vi "System_Main.vi"() -> ()   [LabVIEW 2015, in "System.lvclass"]
uses:
  Classes/System/System.lvclass
  Classes/System/System.lvclass/System.ctl
  Classes/AssetInterface/Interface_Asset.lvclass
  Classes/DispatchInterface/Interface_Dispatch.lvclass
  Classes/TagBus/TagBus.lvclass
panel:
  out "Tag Values":dbl[](array[numeric])
  out "Tag Names":string[](array[string])
  in  "stop":bool
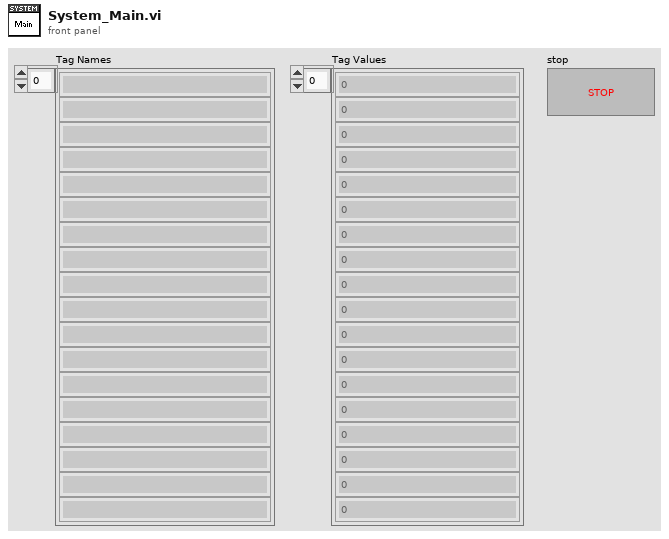
[diagram p1: front panel]
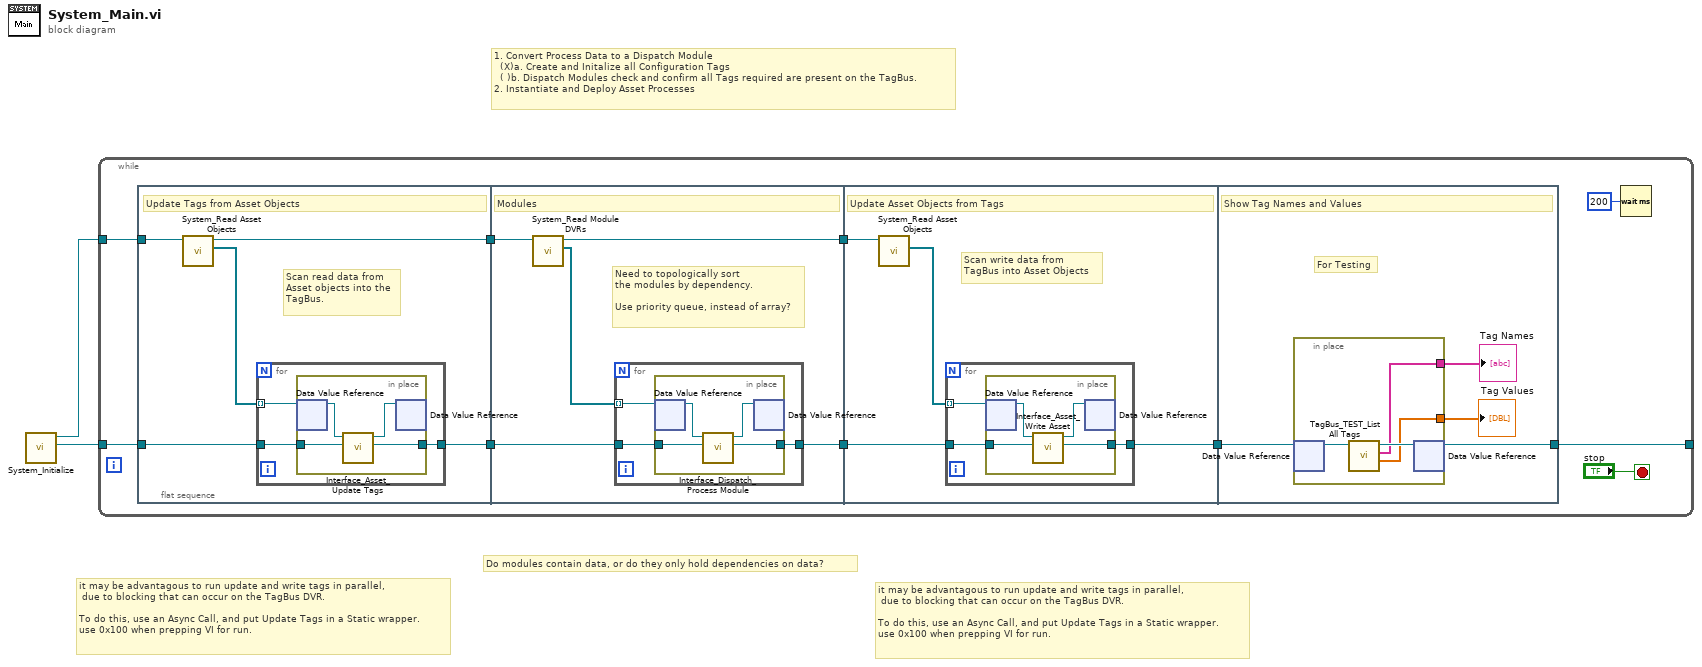
[diagram p0: block diagram]
diagram:
  # "Do modules contain data, or do they only hold dependencies on data?"
  # "it may be advantagous to run update and write tags in parallel,\n due to blocking that can occur on the TagBus DVR.\n\nTo do this, use an Async Call, and put Update Tags in a Static wrapper.\nuse 0x100 when prepping VI for run."
  # "it may be advantagous to run update and write tags in parallel,\n due to blocking that can occur on the TagBus DVR.\n\nTo do this, use an Async Call, and put Update Tags in a Static wrapper.\nuse 0x100 when prepping VI for run."
  # "1. Convert Process Data to a Dispatch Module\n  (X)a. Create and Initalize all Configuration Tags\n  ( )b. Dispatch Modules check and confirm all Tags required are present on the TagBus.\n2. Instantiate and Deploy Asset Processes"
  n1 = call "System_Initialize.vi"() -> ("TagBus DVR"=w1:refnum<data-value>, "System DVR out"=w2:refnum<data-value>)  [unwired: 10 in]
  n2 = while {
    tunnel: w1 -> [w8]
    tunnel: w2 -> [w10]
    tunnel: [w9] -> _
    stop <- "stop" stop-if-true
    n3 = flat-sequence {
      tunnel: w10 -> [w17]
      tunnel: [w15] -> w7
      tunnel: w8 -> [w14]
      tunnel: [w13] -> w6
      tunnel: w7 -> [w29]
      tunnel: [w28] -> w5
      tunnel: w6 -> [w26]
      tunnel: [w25] -> w4
      tunnel: w5 -> [w40]
      tunnel: w4 -> [w37]
      tunnel: [w38] -> w3
      tunnel: [w50] -> w9
      tunnel: w3 -> [w51]
      frame #0 {
        # "Scan read data from\nAsset objects into the\nTagBus."
        # "Update Tags from Asset Objects"
        n4 = call "System_Read Asset Objects.vi"("data value reference"=w17) -> ("Asset DVR Array"=w16:refnum<data-value>[], "data value reference out"=w15:refnum<data-value>)  [unwired: 9 in]
        n5 = for {
          tunnel: w16 -> [w18] mode=indexing
          tunnel: w14 -> [w20]
          tunnel: [w19] -> w13
          n6 = in-place {
            in-place-border: w20 -> [w24]
            in-place-border: [w23] -> w19
            n7 = in-place-dvr #1(w18) -> (w22:refnum<class "Interface_Asset.lvclass">)  [unwired: 1 out]
            n8 = call-dynamic "Interface_Asset_Update Tags.vi"("TagBus DVR"=w24, "Asset_Interface in"=w22) -> ("TagBus DVR out"=w23:refnum<data-value>, "Asset_Interface out"=w21:refnum<class "Interface_Asset.lvclass">)  [unwired: 7 in, 1 out]
            n9 = in-place-dvr #1(w21) -> ()  [unwired: 2 out]
          }
        }
      }
      frame #1 {
        # "Need to topologically sort\nthe modules by dependency.\n\nUse priority queue, instead of array?"
        # "Modules"
        n10 = call "System_Read Module DVRs.vi"("Data Value Reference in"=w29) -> ("Dispatch Module DVR Array"=w27:refnum<data-value>[], "Data Value Reference out"=w28:refnum<data-value>)  [unwired: 9 in]
        n11 = for {
          tunnel: w27 -> [w30] mode=indexing
          tunnel: w26 -> [w32]
          tunnel: [w31] -> w25
          n12 = in-place {
            in-place-border: w32 -> [w34]
            in-place-border: [w33] -> w31
            n13 = in-place-dvr #2(w30) -> (w36:refnum<class "Interface_Dispatch.lvclass">)  [unwired: 1 out]
            n14 = call-dynamic "Interface_Dispatch_Process Module.vi"("TagBus DVR"=w34, "Interface_Dispatch in"=w36) -> ("TagBus DVR out"=w33:refnum<data-value>, "Interface_Dispatch out"=w35:refnum<class "Interface_Dispatch.lvclass">)  [unwired: 7 in, 1 out]
            n15 = in-place-dvr #2(w35) -> ()  [unwired: 2 out]
          }
        }
      }
      frame #2 {
        # "Scan write data from\nTagBus into Asset Objects"
        # "Update Asset Objects from Tags"
        n16 = call "System_Read Asset Objects.vi"("data value reference"=w40) -> ("Asset DVR Array"=w39:refnum<data-value>[])  [unwired: 9 in, 1 out]
        n17 = for {
          tunnel: w39 -> [w41] mode=indexing
          tunnel: w37 -> [w43]
          tunnel: [w42] -> w38
          n18 = in-place {
            in-place-border: w43 -> [w45]
            in-place-border: [w44] -> w42
            n19 = in-place-dvr #3(w41) -> (w46:refnum<class "Interface_Asset.lvclass">)  [unwired: 1 out]
            n20 = call-dynamic "Interface_Asset_Write Asset.vi"("TagBus DVR"=w45, "Asset_Interface in"=w46) -> ("TagBus DVR out"=w44:refnum<data-value>, "Asset_Interface out"=w47:refnum<class "Interface_Asset.lvclass">)  [unwired: 7 in, 1 out]
            n21 = in-place-dvr #3(w47) -> ()  [unwired: 2 out]
          }
        }
      }
      frame #3 {
        # "For Testing"
        # "Show Tag Names and Values"
        n22 = in-place {
          in-place-border: [w53] -> w49
          in-place-border: [w52] -> w48
          n23 = in-place-dvr #4(w51) -> (w55:refnum<class "TagBus.lvclass">)  [unwired: 1 out]
          n24 = call "TagBus_TEST_List All Tags.vi"("TagBus in"=w55) -> ("values"=w52:dbl[], "Double"=w53:string[], "TagBus out"=w54:refnum<class "TagBus.lvclass">)  [unwired: 7 in, 1 out]
          n25 = in-place-dvr #4(w54) -> (w50:refnum<data-value>)  [unwired: 1 out]
        }
        "Tag Names" <- w49
        "Tag Values" <- w48
      }
    }
    n26 = Wait (ms)(milliseconds to wait=u32 200) -> ()  [unwired: 1 out]
  }
